vi "cal_pressure.vi"(9 "calibration pressure":sgl format="%_1f", 10 "Address":u16, 11 "VISA resource name":refnum<visa-resource-name>) -> ()   [LabVIEW 2014]
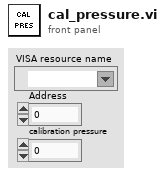
[diagram p1: front panel]
types:
  T1 = enum16{"big-endian, network order", "native, host order", "little-endian"}
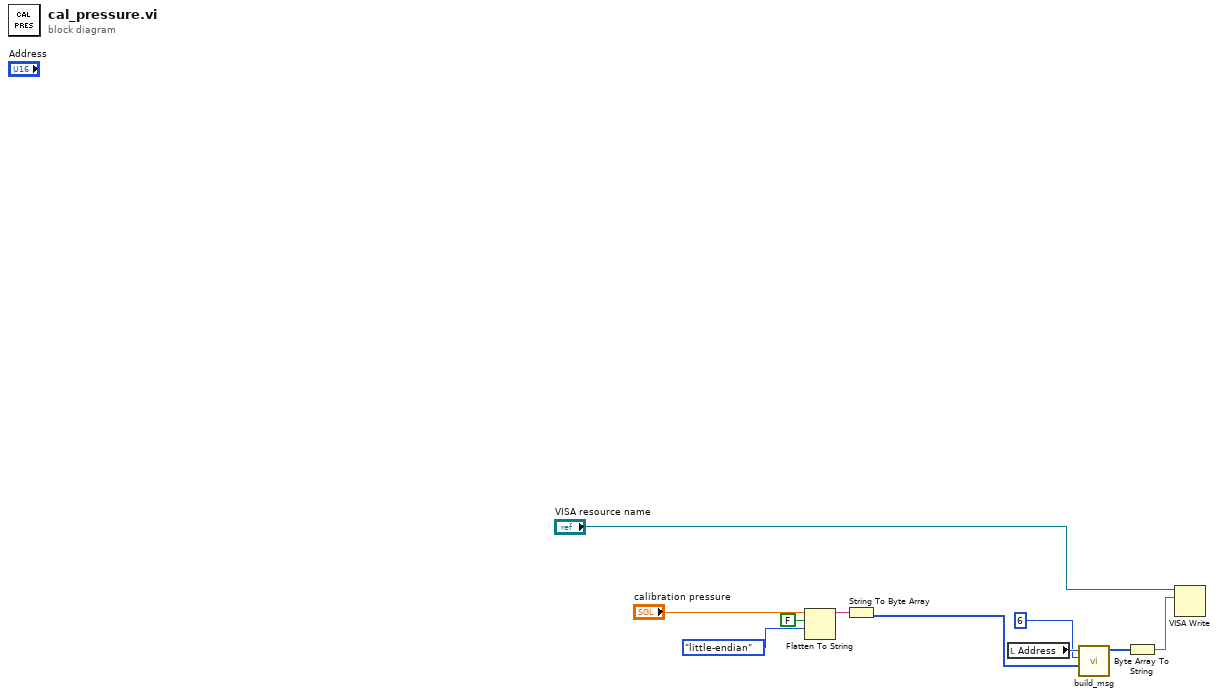
[diagram p0: block diagram]
diagram:
  n1 = Flatten To String(anything="calibration pressure", prepend array or string size? (T)=FALSE, byte order (0:big-endian, network order)=T1."little-endian") -> (data string=w2:string)  [unwired: 1 in, 2 out]
  n2 = String To Byte Array(string=w2) -> (unsigned byte array=w1:u8[])
  n3 = local read "Address"() -> (w10:u16)
  n4 = call "build_msg.vi"("data"=w1, "ID"=u16 6, "Address"=w10) -> ("msg"=w8:u8[])  [unwired: 8 in]
  n5 = Byte Array To String(unsigned byte array=w8) -> (string=w7:string)
  n6 = VISA Write(VISA resource name="VISA resource name", write buffer=w7) -> ()  [unwired: 1 in, 3 out]
